vi "TCP Server Listener Process.vi"() -> ()   [LabVIEW 2020, in "JKI TCP Server.lvclass"]
uses:
  JKI TCP Server.lvclass
  JKI TCP Server.lvclass/JKI TCP Server.ctl
panel:
  in  "TCP Server":refnum<class "JKI TCP Server.lvclass">
  # "This VI Must Be Reentrant"
  # "Copyright © 2004-2008 JKI. All rights reserved.\n\nAuthor: Jim Kring [jim.kring@jameskring.com]\n\nThis library is provided \"AS IS\" ,WITHOUT WARRANTIES OR \nCONDITIONS OF ANY KIND, either express or implied.\n\nJames Kring, Inc. -- http://www.jameskring.com"
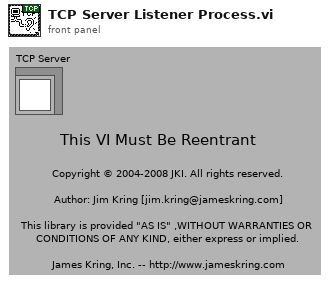
[diagram p1: front panel]
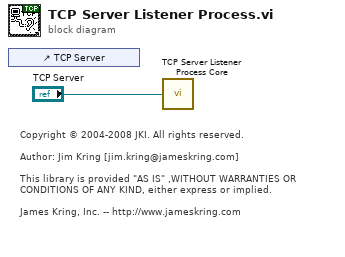
[diagram p0: block diagram]
diagram:
  # "Copyright © 2004-2008 JKI. All rights reserved.\n\nAuthor: Jim Kring [jim.kring@jameskring.com]\n\nThis library is provided \"AS IS\" ,WITHOUT WARRANTIES OR \nCONDITIONS OF ANY KIND, either express or implied.\n\nJames Kring, Inc. -- http://www.jameskring.com"
  n1 = control-ref of="TCP Server"() -> ()  [unwired: 1 out]
  n2 = call "TCP Server Listener Process Core.vi"("TCP Server RefNum"="TCP Server") -> ()
